vi "AlliGator Lifetime Variance Maps Calculation.vi"(7 "AlliGator Ctrl Refnums":T3, 8 "error in (no error)":errorcluster, 9 "Function Parameters":T1={"Function"=enum."Single-Exponential", "Amplitude"=0.0, "Exponent/Scale"=0.0, "Baseline"=0.0, "Residuals SDV"=0.0, "Minimum CL (%)"=1.0, "Analysis Type"=enum."Reference", "Bootstrap SDV x Scale Factor"=1.0, "Residuals SDV x Scale Factor"=1.0, "Low CL Percentile to Reject (%)"=1.0} {"Low CL Percentile to Reject (%)" min=0.0 max=100.0; "Residuals SDV x Scale Factor" min=0.0 max=100.0; "Bootstrap SDV x Scale Factor" min=0.0 max=100.0; "Minimum CL (%)" min=1.0}, 11 "AlliGator IV DVR in":refnum<data-value>) -> (0 "error out":errorcluster, 1 "Parameter Map Names":string[](array[string]), 2 "New Parameter Set Name":string, 3 "AlliGator IV DVR out":refnum<data-value>, 4 "Message":string)   [LabVIEW 2021, in "AlliGator Decay Fit Parameter Map.lvlib"]
uses:
  AlliGator Decay Fit Parameter Map.lvlib
  Internal Variables/AlliGator Internal Variables v2.ctl
  <vilib>/vision/Image Controls.llb/IMAQ Image.ctl
  Internal Variables/AlliGator Gate Image Set.ctl
  Files/AlliGator FLI Dataset Type.ctl
  Files/AlliGator Data Series Type.ctl
  Dual-Channel Datasets/AlliGator Dataset Channel.ctl
  Settings/AlliGator Gate Arithmetic.ctl
  Source Image/AlliGator Displayed Image.ctl
  Image/Named ROI Description.ctl
  Phasor Graph/AlliGator Decay Metadata v3.ctl
  Decay Analysis/Decay Preprocessing/AlliGator Decay Background Subtraction Info.ctl
  Decay Analysis/Decay Preprocessing/AlliGator Baseline Subtraction Method.ctl
  Graphs/XY Graph/XY Graph Plot Shift Parameters.ctl
  Graphs/XY Graph/XY Graph Plot Shift Method.ctl
  Decay Analysis/Decay Preprocessing/AlliGator Decay Extrapolation Parameters.ctl
  Phasor/Calibration Phasor (m, phi).ctl
  Phasor/Phasor Reference Series.ctl
  Phasor/Phasor Calibration Map v2.ctl
  Phasor/Phasor (g, s).ctl
  Phasor Graph/AlliGator Raw Phasor Plot Data v5.ctl
  Phasor/Phasor Standard Deviation Options.ctl
  Phasor Plot/AlliGator Phasor Multi-Harmonic Data.ctl
  Phasor/Phasor Harmonic Data.ctl
  AlliGator Decay Fit Options & Parameters v4.ctl
  Fits/IRF(X)PSED/Decay Fit Options v4.ctl
  Fits/Decay Convolution/Decay Model.ctl
  Fits/Residual Type.ctl
  Fits/IRF(X)PSED/Fit Weights Type v2.ctl
  Fits/Non-linear Fitting Method v2.ctl
  Fits/Fit Calculation Method.ctl
  Fits/Non-linear Fitting Algorithm.ctl
  Decay Analysis/Decay Fit/AlliGator Decay Fit Parameter Constraints 2.ctl
  Fits/IRF(X)PSED/Decay Fit Parameters In List.ctl
  Fits/IRF(X)PSED/MLE Baseline Offset Type.ctl
  Decay Analysis/Decay Preprocessing/AlliGator Decay Preprocessing Parameters.ctl
  Fits/IRF(X)PSED/Decay Fit Parameters & Derived Quantities List v2.ctl
  Fits/IRF(X)PSED/Decay Fit Result Constraint.ctl
  AlliGator Parameter Maps Data.ctl
  GUI/AlliGator Ctrl Refnums.ctl
  GUI/AlliGator Other Ctrl Refnums.ctl
  GUI/AlliGator State Indicator.ctl
  GUI/AlliGator Main Window Tabs.ctl
  GUI/AlliGator Phasor Plot Ctrl Refnums.ctl
  GUI/AlliGator Phasor Graph Ctrl Refnums.ctl
  Phasor/Phasor Calibration Type.ctl
  GUI/AlliGator Dataset Ctrl Refnums.ctl
  GUI/AlliGator Registered Events Ctrl Refnums.ctl
  GUI/AlliGator Image Histogram Control Refnums.ctl
  Histograms/Linear Histogram Options.ctl
  Histograms/Histogram Bin Option.ctl
  Histograms/Histogram Bin Position.ctl
  AlliGator Decay Fit Map Control Refnums.ctl
  Parameter Map/AlliGator Parameter Map Control Refnums.ctl
  AlliGator Function Parameters.ctl
  AlliGator CV(tau) Model Function.ctl
  Globals, Variables, Constants/AlliGator Variables List.ctl
  Camera Noise Influence on Lifetime/Lifetime Variance Data.ctl
  Variant/Variant to Data/Variant to U16.vi
  Variant/Variant to Data/Variant to I32.vi
  <vilib>/Utility/error.llb/Error Cluster From Error Code.vi
  <vilib>/ErrorRing/Error Ring.xnode
  Globals, Variables, Constants/AlliGator Globals, Variables & Constants.lvlib
  Variant/Variant to Data/Variant to Data.lvlib
  Files/AlliGator Files.lvlib
  Fits/Fits.lvlib
  Image/Image.lvlib
  Lifetime & Other Parameters/AlliGator Lifetime & Other Parameters.lvlib
  Strings/Strings.lvlib
  Time/Time.lvlib
  Variant/Variant.lvlib
  Phasor/Phasor.lvlib
  Decay Analysis/Decay Preprocessing/AlliGator Decay Preprocessing.lvlib
  Phasor Graph/AlliGator Phasor Graph.lvlib
  Internal Variables/AlliGator Internal Variables.lvlib
  Phasor Plot/AlliGator Phasor Plot.lvlib
  Source Image/AlliGator Source Image.lvlib
  Decay Analysis/Decay Fit/AlliGator Decay Fit.lvlib
  Settings/AlliGator Settings.lvlib
  Dual-Channel Datasets/AlliGator Dual-Channel Datasets.lvlib
  GUI/AlliGator GUI.lvlib
  Histograms/Histogram Window.lvlib
  Graphs/XY Graph/XY Graph Add-Ons.lvlib
  Parameter Map/AlliGator Parameter Map.lvlib
panel:
  out "CPU (s)":dbl
  # "see the AlliGator License on the block diagram (Ctrl+E or Window:Show Block Diagram)"
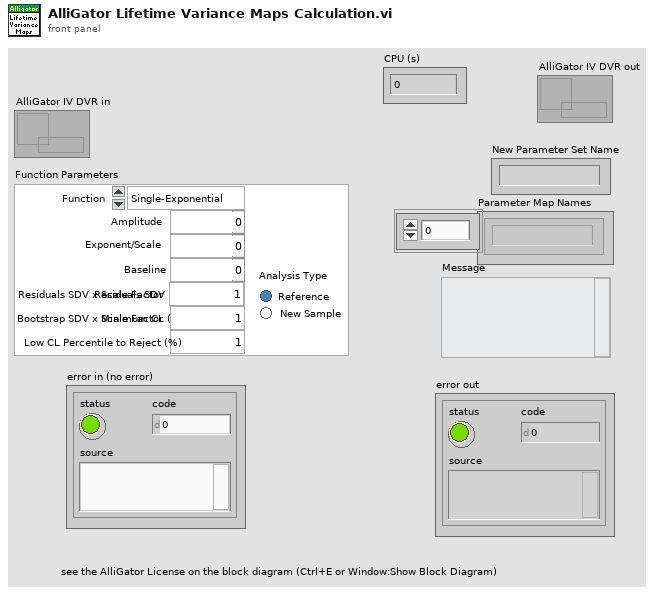
[diagram p1: front panel]
types:
  T1 = typedef "AlliGator Decay Fit Parameter Map.lvlib/AlliGator Function Parameters.ctl" = cluster{"Function":T2, "Amplitude":dbl, "Exponent/Scale":dbl, "Baseline":dbl, "Residuals SDV":dbl, "Minimum CL (%)":dbl, "Analysis Type":enum32{"Reference", "New Sample"}, "Bootstrap SDV x Scale Factor":dbl, "Residuals SDV x Scale Factor":dbl, "Low CL Percentile to Reject (%)":dbl}
  T2 = typedef "AlliGator Lifetime & Other Parameters.lvlib/AlliGator CV(tau) Model Function.ctl" = enum16{"Single-Exponential", "Power Law"}
  T3 = typedef "AlliGator GUI.lvlib/AlliGator Ctrl Refnums.ctl" = cluster{"Other AlliGator Ctrl Refnums":T4, "Phasor Plot Ctrl Refnums":T5, "Phasor Graph Ctrl Refnums":T6, "Dataset Control Refnums":T7, "Registered Events Ctrl Refnums":T8, "Image Histogram Ctrl Refnums":T9, "Decay Fit Map Ctrl Refnums":T10, "Parameter Map Ctrl Refnums":T11}
  T4 = typedef "AlliGator GUI.lvlib/AlliGator Other Ctrl Refnums.ctl" = cluster{"State Indicators":refnum<vi>, " Progress Bar":refnum<vi>, "Decay Graph Active":refnum<vi>, "Decay Statistics Bin":refnum<vi>, "Time Step":refnum<vi>, "Use File Timestamp":refnum<vi>, "Tab Control":refnum<vi>, "CPU":refnum<vi>, "Abort Fit":refnum<vi>, "Dataset File/Folder Path":refnum<vi>, "Abort ROI Creation":refnum<vi>, "Event LED":refnum<vi>, "Dataset File/Folder Path 2":refnum<vi>, "Dataset File/Folder Path 3":refnum<vi>, "Dataset File/Folder Path 4":refnum<vi>, "Dataset File/Folder Path 5":refnum<vi>, "Dataset File/Folder Path 6":refnum<vi>, "Dataset File/Folder Path 7":refnum<vi>, "Dataset File/Folder Path 8":refnum<vi>, "Dataset File/Folder Path 9":refnum<vi>, "Dataset File/Folder Path 10":refnum<vi>, "Dataset File/Folder Path 11":refnum<vi>}
  T5 = typedef "AlliGator GUI.lvlib/AlliGator Phasor Plot Ctrl Refnums.ctl" = cluster{"Phasor Ratio":refnum<vi>, "Modulus Lifetime":refnum<vi>, "Phasor at cursor (m, phi)":refnum<vi>, "Phase Lifetime":refnum<vi>, "Phasor at cursor (g, s)":refnum<vi>, "Phasor Plor Average Lifetime":refnum<vi>, "Phasor Plot Active":refnum<vi>, "Save Phasor Plot":refnum<vi>, "Image Overlay Color":refnum<vi>, "Phasor Plot Color Scale":refnum<vi>, "Reference 1 Button":refnum<vi>, "Reference 2 Button":refnum<vi>, "True Phasor Plot Value":refnum<vi>}
  T6 = typedef "AlliGator GUI.lvlib/AlliGator Phasor Graph Ctrl Refnums.ctl" = cluster{"Phasor Ratio":refnum<vi>, "Modulus Lifetime":refnum<vi>, "Phasor at cursor (m, phi)":refnum<vi>, "Phase Lifetime":refnum<vi>, "Phasor at cursor (g, s)":refnum<vi>, "Phasor Graph Average Lifetime":refnum<vi>, "Phasor Graph Active":refnum<vi>, "Save Phasor Graph":refnum<vi>, "Phasor Frame Slide":refnum<vi>, "Single Step Phasor":refnum<vi>, "Calibration Type":refnum<vi>, "Show Line":refnum<vi>, "Phase Lifetime 1":refnum<vi>, "Phase Lifetime 2":refnum<vi>, "Phasor Graph Frequency":refnum<vi>, "Phasor Reference 1 Control":refnum<vi>, "Phasor Reference 2 Control":refnum<vi>, "Calibration Lifetime":refnum<vi>, "Phase Lifetime SDV":refnum<vi>, "Average Lifetime SDV":refnum<vi>, "Phasor Ratio SDV":refnum<vi>, "Modulus Lifetime SDV":refnum<vi>}
  T7 = typedef "AlliGator GUI.lvlib/AlliGator Dataset Ctrl Refnums.ctl" = cluster{"Current Data":refnum<vi>, "Gate Image Slide":refnum<vi>, "Time Point Slide":refnum<vi>, "Current Time Stamp":refnum<vi>, "Save Image":refnum<vi>, "Displayed Image":refnum<vi>, "Overlay Mode":refnum<vi>, "Phasor Overlay Color":refnum<vi>, "Image Color Scale":refnum<vi>, "Use ROI as Search Area":refnum<vi>, "Source Image ROI Color":refnum<vi>, "True Pixel Value":refnum<vi>}
  T8 = typedef "AlliGator GUI.lvlib/AlliGator Registered Events Ctrl Refnums.ctl" = cluster{"Time Point Slider":refnum<vi>, "Phasor Plot Display Range":refnum<vi>, "Decay Graph":refnum<vi>, "Decay Statistics Graph":refnum<vi>, "Intensity Time Trace":refnum<vi>, "Phasor Graph":refnum<vi>, "Phasor Ratio Graph":refnum<vi>, "Lifetime Graph":refnum<vi>, "Phasor Plot Display":refnum<vi>, "Source Image Display":refnum<vi>, "Decay Fit Parameter Map Display Range":refnum<vi>, "Decay Fit Parameter Map Display":refnum<vi>, "Parameter Map Display Range":refnum<vi>, "Parameter Map Display":refnum<vi>, "Phasor Plot Display Range":refnum<vi>}
  T9 = typedef "AlliGator GUI.lvlib/AlliGator Image Histogram Control Refnums.ctl" = cluster{"Image Histogram":refnum<vi>, "Image Histogram Options":refnum<vi>, "Image Histogram Active":refnum<vi>, "Image Histogram Upper Percentile":refnum<vi>, "Image Histogram Lower Percentile":refnum<vi>, "Auto-Adjust Contrast":refnum<vi>}
  T10 = typedef "AlliGator Decay Fit Parameter Map.lvlib/AlliGator Decay Fit Map Control Refnums.ctl" = cluster{"Decay Fit Parameter Map Color Scale":refnum<vi>, "Decay Fit Parameter":refnum<vi>, "Max Parameter":refnum<vi>, "Min Parameter":refnum<vi>, "Decay Fit Parameter Map Display":refnum<vi>, "Decay Fit Parameter Map Display Range":refnum<vi>, "Decay Parameter Map X":refnum<vi>, "Decay Parameter Map Y":refnum<vi>, "Decay Parameter Map Value":refnum<vi>}
  T11 = typedef "AlliGator Parameter Map.lvlib/AlliGator Parameter Map Control Refnums.ctl" = cluster{"Parameter Map Color Scale":refnum<vi>, "Map Parameter":refnum<vi>, "Max Parameter":refnum<vi>, "Min Parameter":refnum<vi>, "Parameter Map Display":refnum<vi>, "Parameter Map Display Range":refnum<vi>, "Parameter Map Set":refnum<vi>, "Parameter Map X":refnum<vi>, "Parameter Map Y":refnum<vi>, "Parameter Map Value":refnum<vi>}
  T12 = typedef "AlliGator Globals, Variables & Constants.lvlib/AlliGator Variables List.ctl" = enum16{"---- GUI ----", "GUI:Initialization Status", "GUI:State Indicators Refnum", "GUI:Original AlliGator Menu Items", "GUI:Current Action Loop State", "GUI:Script in progress", "GUI:Playback", "GUI:Loop Playback", "GUI:Search ROI Used", "GUI:Search ROI", "Decay Graph Max Legend Size", "Intensity Graph Max Legend Size", "Decay Statistics Graph Max Legend Size", "Phasor Graph Max Legend Size", "Phasor Ratio Graph Max Legend Size", "Lifetime Graph Max Legend Size", "---- Files ----", "Files:Export Dataset Frames as Individual Files", "Files:Show Batch Export Help Balloons", "Files:Frames in Dataset", "Files:ptu File Frame Start Indices", "Files:Current Frame in Dataset", "Files:Current Frame Timestamp", "Files:Dataset Loaded", "Files:Dataset Metadata", "Files:Dataset Channel", "Files:Dataset Data Description", "Files:Background Dataset Metadata", "Files:Background Dataset Channel", "Files:Background Dataset Data Description", "Files:Background File Subtraction", "Files:Background File Path", "Files:Background File Pile-up Correction", "Files:Background File Pixel Well Capacity", "Files:Background File Scaling Factor", "Files:Current Dataset Load Settings", "Files:Dataset Path", "Files:ICCD-specific Information", "Files:Macrotime Gate Separation", "------ Python Plugins ------", "Python Plugins:Information", "Python Plugins:Python Session", "Python Plugins:Valid Python Session?", "---- Source Image ----", "Source Image:ROIs", "Source Image:Current ROI", "Source Image:ROI Event Refnum", "X_Source Image:Display Range", "X_Source Image:Palette Information", "X_Source Image:Type of Displayed Image", "X_Time Gate Slider", "Source Image:Palette List", "Source Image:Scale", "Source Image:ROI Overlay Color", "Source Image:Overlay to Erase", "Source Image:Is Displayed Image Accumulated", "Source Image:White Light Image Modified", "Source Image:Mask Image Modified", "---- Image Profile Window ----", "Image Profile:Window Event Refnum", "Image Profile:IntensityType", "Image Profile:Intensity Average Type", "Image Profile:Intensity-weighted SDV", "Image Profile:Box Profile Type", "Image Profile:Window Open", "Image Profile:Plotted Fit Parameter", "------ Phasor Graph -------", "Phasor Graph:Show Line", "---- Phasor Plot ---", "Phasor Plot:Parameters Changed", "Phasor Plot:FLI Dataset Modified since last Calculation", "Phasor Harmonics Data", "Selected Phasor Harmonics", "Phasor Harmonic Manager Event Refnum", "Phasor Plot:ROIs", "Phasor Plot:Current ROI", "Phasor Plot:ROI Event Refnum", "Phasor Plot:Image Reference Points", "Phasor Plot:Computed", "Phasor Plot:Palette Information", "Phasor Plot:Palette List", "Phasor Plot:Phasor Ratio Palette Information", "Phasor Plot:Phasor Ratio Palette List", "Phasor Plot:Image Scale", "Phasor Plot:Image Overlay to Erase", "Phasor Plot:Image Elements to Update", "Phasor Plot:Current Calculation Parameters", "Phasor Plot:Current Calibration Options", "Phasor Plot:Reset Cumulated Phasor Plot", "Phasor Plot:Reference 1", "Phasor Plot:Lifetime Reference 1", "Phasor Plot:Reference 1 Frequency", "Phasor Plot:Reference 2", "Phasor Plot:Lifetime Reference 2", "Phasor Plot:Reference 2 Frequency", "---- Decay Analysis ----", "Number of Selected Decays to Fit", "LS Fit Results", "LAR Fit Results", "BS Fit Results", "Last Decay Max - Min", "Best Fit Parameters", "Best Fit Parameter Names", "Actual Size X", "Actual Size Y", "Binning X", "Binning Y", "Actual # Gates", "Dataset Number", "Gates to...", "Gates Skipped", "Gates to keep", "Gate Step", "Gate Separation", "Reversed Gates", "Pile-up Correction", "Pixel Well Capacity", "Background Subtracted", "Background Subtraction Method", "Background Definition Range", "Background File (deprecated)", "Number of Dataset Accumulated", "Array of Accumulated Dataset Paths", "Do Averaged Datasets", "Destination File Path", "Process Plot Target", "Use 1/D as Phasor Frequency", "---- Decay Fit Parameter Map -----", "Decay Fit Parameter Map:Palette Information", "Decay Fit Parameter Map:Palette List", "Decay Fit Parameter Map:X Resolution", "Decay Fit Parameter Map:Y Resolution", "Decay Fit Parameter Map:Use Decay Fit Result Constraints", "Decay Fit Parameter Map:Decay Fit Result Constraints", "Decay Fit Parameter Map:Decay Fit Result Constraints Applied", "---- Parameter Map ----", "Parameter Map:Palette Information", "Parameter Map:Palette List", "------- Local Decay Window ---------", "Local Decay Graph Window:Event Refnum", "Local Decay Graph Window:Use normalized IRF for convolution", "----- Miscellaneous ----", "Misc:Skippable Dialog Windows Status"}
  T13 = typedef "Image.lvlib/Named ROI Description.ctl" = cluster{"ROI Descriptor":T14, "ROI Name":string, "Overlay Color":u32}
  T14 = typedef "ROI Descriptor" = cluster{"Global Rectangle":i32[], "Contours":cluster{"ID":enum32{"External", "Internal"}, "Type":u32, "Coordinates":i32[]}[]}
  T15 = typedef "Fits.lvlib/Decay Fit Parameters & Derived Quantities List v2.ctl" = enum16{"Offset", "Baseline", "A_1", "tau_1", "A_2", "tau_2", "<tau>_a", "f1_a", "f2_a", "<tau>_i", "f1_i", "f2_i", "-", "R^2", "Chi^2"}
  T16 = typedef "AlliGator Decay Fit Parameter Map.lvlib/AlliGator Parameter Maps Data.ctl" = cluster{"Map Set Name":string, "[Parameter Names]":string[], "[[Parameters]]":dbl[][], "[[Parameter SDVs]]":dbl[][], "Decay Array Time Axis":dbl[], "[[IRFs]]":dbl[][], "IRF Array Time Axis":dbl[], "X Resolution":i32, "Y Resolution":i32, "Intensity Array":dbl[]}
  T17 = typedef "AlliGator Decay Fit Parameter Map.lvlib/Lifetime Variance Data.ctl" = cluster{"ROI Name":string, "Intensity Array":sgl[], "Lifetime Array":dbl[], "Coordinate Array":cluster{"X":i32, "Y":i32}[], "I Slice Bin Boundaries":dbl[], "Sliced <tau>":dbl[], "Sliced SDV(<tau>)":dbl[], "Sliced CV(<tau>)":dbl[], "Sliced #Elements":i32[], "I Slice <I>":dbl[], "Sliced CV SDV(<tau>)":dbl[]}
  T18 = typedef "AlliGator Internal Variables.lvlib/AlliGator Internal Variables v2.ctl" = cluster{"----------------------------- Images -----------------------------":u8, "Displayed Image":T19, "White Light Image":T19, "Mask Image":T19, "ROI Mask Image":T19, "Current Dataset Images 1":T20, "Background Dataset Images 1":T20, "Current Dataset Images 2":T20, "Background Dataset Images 2":T20, "Current Dataset Arithmetic Images":T20, "Accumulated Dataset Images 1":T20, "Accumulated Dataset Images 2":T20, "Accumulated Dataset Arithmetic Images":T20, "----------------------------- File Paths -----------------------------":u8, "Phasor Plot Image":T19, "Decay Fit Parameter Map Image":T19, "Parameter Map Image":T19, "Single Data Point Path":path, "White Light Image Path":path, "Mask Image Path":path, "Time-Series Folder":path, "[Time-Series Paths]":path[], "----------------------------- FLI Dataset -----------------------------":u8, "Current Dataset":i32, "Single Dataset Type":T21, "Current Folder":string, "AlliGator Data Series Type":T22, "# Datasets":i32, "Dual-Channel Dataset":bool, "Selected Channel Name":string, "Dataset Channel":T23, "Channel Arithmetic":T24, "Dual-Channel Background Dataset":bool, "Background Channel":T23, "Dual-Channel Accumulated Dataset":bool, "Start Time":dbl, "[Time-Series Timestamps]":dbl[], "[Intensity Corrections]":dbl[], "Time Series Script":bool, "Type of Displayed Image":T25, "Gate Image Slide":u16, "# Gates":i32, "ROIs":T13[], "----------------------------- Decays -----------------------------":u8, "ROI Decay":cluster{"t Array":dbl[], "I Array":dbl[]}, "Valid Decay":bool, "Decay  Metadata":T26, "Reference Decay Plot Name":string, "Reference Decay":cluster{"t Array":dbl[], "I Array":dbl[]}, "Decay Shift Plot":cluster{"Time Stamps":dbl[], "Decay Shifts":dbl[]}, "[Decays Max Values]":sgl[], "[Decays Min Values]":sgl[], "----------------------------- Calibration -----------------------------":u8, "Calibration Phasor":T32, "Calibration Phasor Series":T33, "Phasor Calibration Map":T34, "Calibration Map MD5 Digest":string, "----------------------------- Phasor Graph -----------------------------":u8, "Last Raw Phasor":T35, "Last Calibrated Phasor":T35, "Last Calibrated Phasor SDV":T35, "Phasor Graph:Phasor Plot":cluster{"g Array":dbl[], "s Array":dbl[]}, "Phasor Graph:Phasor SDV Plot":cluster{"g Array":dbl[], "s Array":dbl[]}, "[Phasor Graph:Raw Phasor Plots]":T36[], "Phasor Plot locked to Ref 1":i32, "[Phasor Plot(s) locked to Ref 1]":i32[], "[Phasor Plot(s) locked to Ref 2]":i32[], "[Pixel Phasors]":T35[], "----------------------------- Phasor Plot -----------------------------":u8, "[[Sum Image]]":dbl[][], "[[CSG Phasors]]":csg[][], "[[Valid Pixel?]]":bool[][], "[[Phasor Ratios]]":dbl[][], "[[Average Lifetimes]]":dbl[][], "Amplitude Weighted Average Lifetime":bool, "I/m/phi Dataset":cluster{"I/m/phi Dataset?":bool, "Base Frequency":dbl[unit], "Harmonic Orders":u8[]}, "Multi Phasor Plot Data":T38, "----------------------------- Decay Fit Parameter Map -----------------------------":u8, "Decay Fit Options & Parameters":T40, "Fit Options: Decay Preprocessing Parameters":T51, "Fit Options: Reference Decay":cluster{"t Array":dbl[], "I Array":dbl[]}, "Is Full Image Parameters Map":bool, "Is Single-Pixels Parameters Map":bool, "NLSF Parameters Map X Resolution":i32, "NLSF Parameters Map Y Resolution":i32, "[Single Decay Fit Parameters]":dbl[], "Fit Model":T42, "[[Multiple Decays Fit Parameters]]":dbl[][], "[[Multiple Decays Fit Parameter SDVs]]":dbl[][], "[[IRFs]]":dbl[][], "[ROI Descriptors]":T14[], "IRF Array Time Axis":dbl[], "Decay Array Time Axis":dbl[], "[Decay Fit Parameter Names]":T15[], "[Decay Sum]":dbl[], "Array of Decay Fit Result Constraints":T52[], "Selected ROIs Array":bool[], "----------------------------- Parameter Maps -----------------------------":u8, "[Map Set Names]":string[], "[Parameter Maps]":T16[], "[[User-defined Quantities]]":dbl[][], "User-defined Quantity":string}
  T19 = typedef "IMAQ Image.ctl" = refnum<image>
  T20 = typedef "AlliGator Internal Variables.lvlib/AlliGator Gate Image Set.ctl" = cluster{"SGL Gate Images":T19[], "SGL Sum Image":T19, "SGL Max Image":T19, "SGL Min Image":T19}
  T21 = typedef "AlliGator Files.lvlib/AlliGator FLI Dataset Type.ctl" = enum16{"HDF5 FLI Dataset", "Gate Image Folder", ".sdt FLI Dataset (Becker & Hickl)", ".ptu FLI Dataset (PicoQuant)", "SS1 FLI Dataset", "SS2 FLI Dataset", "I/m/phi Dataset", ".bin FLI Dataset (PicoQuant Binned)", ".bin FLI Dataset (Piccolo Binned)", ".mat FLI Dataset"}
  T22 = typedef "AlliGator Files.lvlib/AlliGator Data Series Type.ctl" = enum16{"Not a Supported Series", "Gate Images Folder Series", "SwissSPAD 2 Dataset Series", "B&H FLI Dataset Series", "PicoQuant PTU FLI Dataset Series", "PicoQuant BIN FLI Dataset Series", "Piccolo hist BIN FLI Dataset Series", "HDF5 FLI Dataset Series"}
  T23 = typedef "AlliGator Dual-Channel Datasets.lvlib/AlliGator Dataset Channel.ctl" = enum16{"G2", "INT"}
  T24 = typedef "AlliGator Settings.lvlib/AlliGator Gate Arithmetic.ctl" = enum16{"None", "INT-G2", "G2/INT*<INT>", "(1 - G2/INT)*<INT>"}
  T25 = typedef "AlliGator Source Image.lvlib/AlliGator Displayed Image.ctl" = enum16{"Single Gate", "Sum of All Gates", "Max of All Gates", "Min of All Gates", "-", "White Ligth Image", "Mask Image"}
  T26 = typedef "AlliGator Phasor Graph.lvlib/AlliGator Decay Metadata v3.ctl" = cluster{"ROI Descriptor":T14, "ROI Center":cluster{"X":i32, "Y":i32}, "Decay Background Subtraction Info":T27, "Decay Reverted":bool, "Decay Smoothened":bool, "Decay Straightened":bool, "Fitted Tau (Decay Straightening)":dbl, "Decay Shift Parameters":T29, "Decay Shifted":bool, "Decay Extrapolated":bool, "Decay Extrapolation Parameters":T31, "Decay Normalized":bool, "Fold Decay":bool, "# Folds":u32}
  T27 = typedef "AlliGator Decay Preprocessing.lvlib/AlliGator Decay Background Subtraction Info.ctl" = cluster{"Laser Period":dbl[unit], "Gate Duration":dbl[unit], "Baseline Subtraction Method":T28, "Background Definition Range":cluster{"Min Gate":dbl[unit], "Max Gate":dbl[unit]}, "Total Intensity w/o Bkgd Subtraction":dbl, "Bkgd-subtracted Intensity (exp)":dbl, "# Data Points":i32, "Background/Gate":dbl, "Fitted Lifetime":dbl[unit], "Bkgd-subtracted Intensity (theo)":dbl}
  T28 = typedef "AlliGator Decay Preprocessing.lvlib/AlliGator Baseline Subtraction Method.ctl" = enum16{"Mean", "Min", "Square Gated Single-Exponential", "File", "Constant"}
  T29 = typedef "XY Graph Add-Ons.lvlib/XY Graph Plot Shift Parameters.ctl" = cluster{"Type":T30, "Shift":dbl[unit], "Threshold":dbl, "Rotate":bool}
  T30 = typedef "XY Graph Add-Ons.lvlib/XY Graph Plot Shift Method.ctl" = enum16{"Default", "CFD", "Threshold", "Cross-Correlation"}
  T31 = typedef "AlliGator Decay Preprocessing.lvlib/AlliGator Decay Extrapolation Parameters.ctl" = cluster{"Additional Points":u32, "Head Fraction":dbl, "Fitted Tau":dbl, "Use Periodicity":bool, "Use Cursors":bool, "Tail Fraction":dbl}
  T32 = typedef "Phasor.lvlib/Calibration Phasor (m, phi).ctl" = cluster{"m":dbl, "phi":dbl, "Phasor Frequency":dbl[unit], "Reference Lifetime":dbl[unit]}
  T33 = typedef "Phasor.lvlib/Phasor Reference Series.ctl" = cluster{"m Array":dbl[], "phi Array":dbl[], "Phasor Frequency":dbl[unit], "Calibration Lifetime":dbl[unit]}
  T34 = typedef "Phasor.lvlib/Phasor Calibration Map v2.ctl" = cluster{"Phasor Frequency":dbl[unit], "Calibration Lifetime":dbl[unit], "ROI Centers":cluster{"X":i32, "Y":i32}[], "ROI Descriptors":T14[], "Map Resolution X":i32, "Map Resolution Y":i32, "z Array":cdb[]}
  T35 = typedef "Phasor.lvlib/Phasor (g, s).ctl" = cluster{"g":dbl, "s":dbl}
  T36 = typedef "AlliGator Phasor Graph.lvlib/AlliGator Raw Phasor Plot Data v5.ctl" = cluster{"Phasor Plot Name":string, "Raw Phasor Plot":T35[], "Phasor Frequency":dbl[unit], "[Decay Metadata]":T26[], "Raw Phasor Plot SDV":T35[], "Phasor SDV Options":T37, "[Calibration Phasor]":T32[], "Intensity Array":dbl[]}
  T37 = typedef "Phasor.lvlib/Phasor Standard Deviation Options.ctl" = cluster{"Compute Estimated SDV":bool, "# Replicas":u32, "Use Estimated Average Phasor":bool}
  T38 = typedef "AlliGator Phasor Plot.lvlib/AlliGator Phasor Multi-Harmonic Data.ctl" = cluster{"Base Frequency":dbl[unit], "# Harmonics":u8, "Harmonic Orders":u8[], "Phasor Plot Settings Checksum":u64, "Phasor Harmonic Data Array":T39[]}
  T39 = typedef "Phasor.lvlib/Phasor Harmonic Data.ctl" = cluster{"Phasor Harmonic Name":string, "Phasor Plot Settings Checksum":u64, "Phasor Frequency":dbl[unit], "Base Frequency":dbl[unit], "Harmonic Order":u8, "Phasor Plot Parameters":string, "Phasor Array [[CSG]]":csg[][], "Dataset File Path":path}
  T40 = typedef "AlliGator Decay Fit Parameter Map.lvlib/AlliGator Decay Fit Options & Parameters v4.ctl" = cluster{"SYNC Period":dbl[unit], "Fit Options":T41, "Fit Parameter Constraints":T48[], "MLE Baseline Offset":dbl, "MLE Baseline Offset Type":T50}
  T41 = typedef "Fits.lvlib/Decay Fit Options v4.ctl" = cluster{"Show Fit Residuals":bool, "Fit Model":T42, "Residual Type":T43, "Max Decay Percentile":dbl, "Min Decay Percentile":dbl, "Show Full Decay":bool, "Weights":T44, "Fitting Method":T45, "Compute Parameter Uncertainties":bool, "Periodic Boundaries":bool, "Model Calculation":T46, "Period":dbl[unit], "Termination Criteria":cluster{"Max Iterations":i32, "Max Function Calls":i32, "Max Time":dbl[unit], "Function Tolerance":dbl, "Parameter Tolerance":dbl, "Gradient Tolerance":dbl, "Min Lambda":dbl, "Max Lambda":dbl, "Initial Tick Count":u32}, "Offset Resolution":dbl[unit], "Use Local IRF":bool, "Fitting Algorithm":T47, "Show Confidence Interval ":bool, "Confidence Level":dbl}
  T42 = typedef "Fits.lvlib/Decay Model.ctl" = enum16{"1-Exponential", "2-Exponentials"}
  T43 = typedef "Fits.lvlib/Residual Type.ctl" = enum16{"Standard", "Normalized", "Reduced"}
  T44 = typedef "Fits.lvlib/Fit Weights Type v2.ctl" = enum16{"Unweighted", "1/Variance (Neyman)", "1/Variance (Pearson)", "Best of All"}
  T45 = typedef "Fits.lvlib/Non-linear Fitting Method v2.ctl" = enum16{"Least Square", "Least Absolute Residual", "Bisquare", "MLE", "-", "Best of All"}
  T46 = typedef "Fits.lvlib/Fit Calculation Method.ctl" = enum16{"Simulation", "Convolution", "Integration"}
  T47 = typedef "Fits.lvlib/Non-linear Fitting Algorithm.ctl" = enum16{"Levenberg-Marquardt", "Trust-Region Dogleg"}
  T48 = typedef "AlliGator Decay Fit.lvlib/AlliGator Decay Fit Parameter Constraints 2.ctl" = cluster{"Fit Parameter":T49, "Min Value":dbl, "Max Value":dbl, "Global":bool, "Used":bool}
  T49 = typedef "Fits.lvlib/Decay Fit Parameters In List.ctl" = enum16{"Offset", "Baseline", "A_1", "tau_1", "A_2", "tau_2"}
  T50 = typedef "Fits.lvlib/MLE Baseline Offset Type.ctl" = enum32{"Absolute", "Percentage"}
  T51 = typedef "AlliGator Decay Preprocessing.lvlib/AlliGator Decay Preprocessing Parameters.ctl" = cluster{"Background Subtraction":bool, "Straighten Decay":bool, "Reverse Gates":bool, "1-Normalized Decay":bool, "Smoothen Decay":bool, "Smoothing Parameter":dbl, "Shift Decay":bool, "Decay Shift Parameters":T29, "Extrapolate Decay":bool, "Additional Points":u32, "Head Fraction":dbl, "Pixel-Normalize Decay":bool, "Use Periodicity":bool, "Use Cursors":bool, "Tail Fraction":dbl, "Use Decay Pre-Processing":bool, "Fold Decay":bool, "# Folds":u32, "[0-1]-Normalized Decay":bool}
  T52 = typedef "Fits.lvlib/Decay Fit Result Constraint.ctl" = cluster{"Fit Parameter":enum16{"Offset", "Baseline", "A_1", "tau_1", "A_2", "tau_2", "<tau>_a", "f1_a", "f2_a", "<tau>_i", "f1_i", "f2_i", "-", "R^2", "Chi^2", "Max Relative Residual", "<Residual ACF>", "Residual ACF SDV", "tau_2/tau_1"}, "Min Value":dbl, "Max Value":dbl, "Use Constraint":bool}
  T53 = typedef "XY Graph Add-Ons.lvlib/XY Graph Sliced Mean & SDV Step Definition.ctl" = cluster{"Axis Start":dbl, "Axis Stop":dbl, "# Steps":i32, "Step Size":dbl, "Step Definition":T54, "Upper Percentile":dbl, "Lower Percentile":dbl, "Min # Data Points/Slice":i32, "Output Abscissa Statistics Plots":bool, "Bin Location":T55, "# Elements":i32, "Bootstrap CV's SDV":bool, "# Replicas":i32}
  T54 = typedef "AlliGator Lifetime & Other Parameters.lvlib/AlliGator Intensity Slice Definition.ctl" = enum32{"# Steps", "Step Size", "# Elements"}
  T55 = typedef "XY Graph Add-Ons.lvlib/XY Graph Sliced CV Abscissa Location.ctl" = enum16{"Left", "Center", "Mean", "Right"}
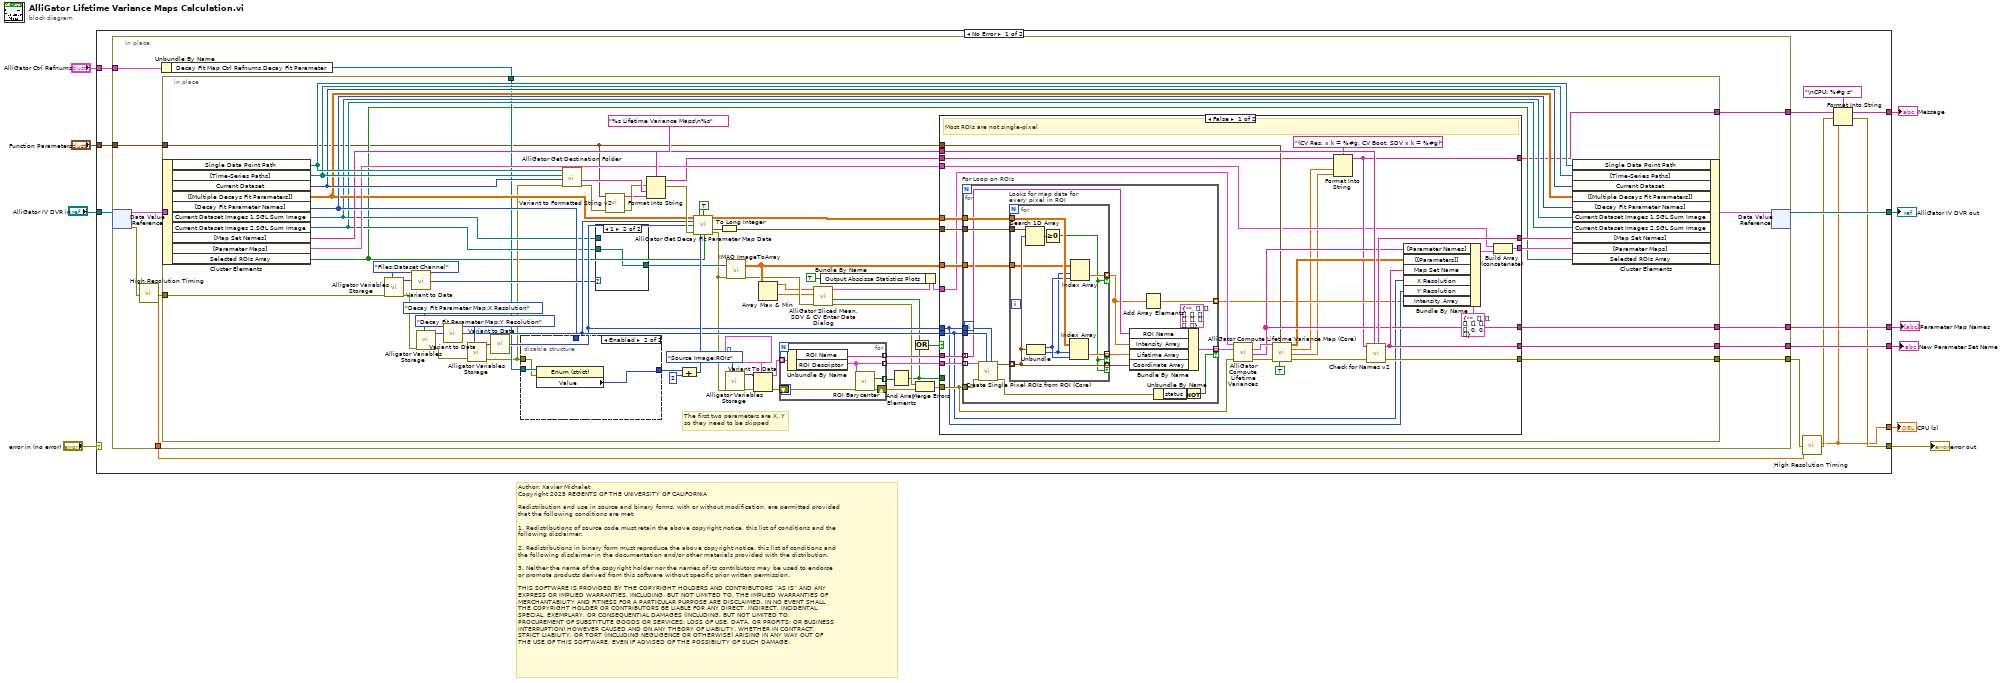
[diagram p0: block diagram]
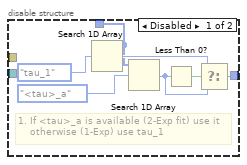
[diagram p2: hidden frame]
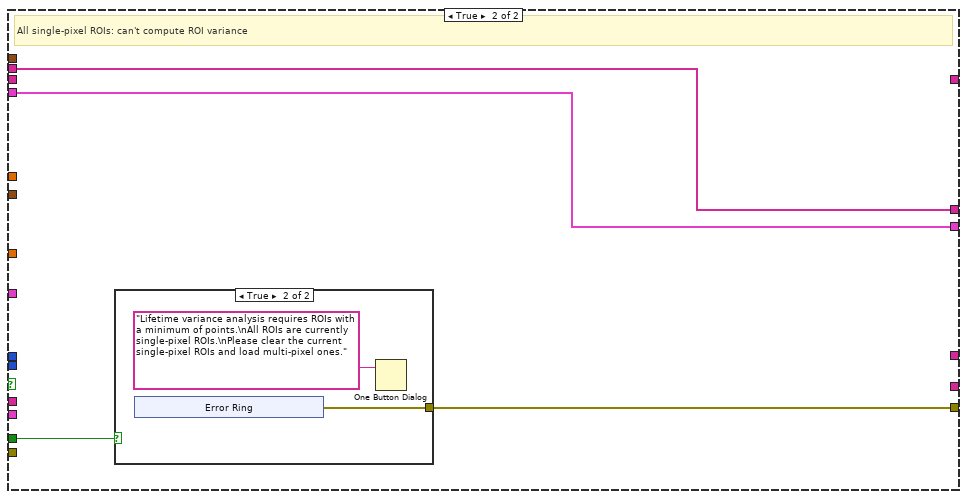
[diagram p3: hidden frame]
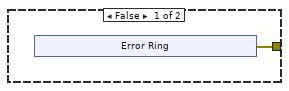
[diagram p4: hidden frame]
diagram:
  # "Author: Xavier Michalet\nCopyright 2025 REGENTS OF THE UNIVERSITY OF CALIFORNIA\n\nRedistribution and use in source and binary forms, with or without modification, are permitted provided\nthat the following conditions are met:\n\n1. Redistributions of source code must retain the above copyright notice, this list of conditions and the\nfollowing disclaimer.\n\n2. Redistributions in binary form must reproduce the above copyright notice, this list of conditions and\nthe following disclaimer in the documentation and/or other materials provided with the distribution.\n\n3. Neither the name of the copyright holder nor the names of its contributors may be used to endorse \nor promote products derived from this software without specific prior written permission.\n\nTHIS SOFTWARE IS PROVIDED BY THE COPYRIGHT HOLDERS AND CONTRIBUTORS “AS IS” AND ANY \nEXPRESS OR IMPLIED WARRANTIES, INCLUDING, BUT NOT LIMITED TO, THE IMPLIED WARRANTIES OF\nMERCHANTABILITY AND FITNESS FOR A PARTICULAR PURPOSE ARE DISCLAIMED. IN NO EVENT SHALL\nTHE COPYRIGHT HOLDER OR CONTRIBUTORS BE LIABLE FOR ANY DIRECT, INDIRECT, INCIDENTAL, \nSPECIAL, EXEMPLARY, OR CONSEQUENTIAL DAMAGES (INCLUDING, BUT NOT LIMITED TO, \nPROCUREMENT OF SUBSTITUTE GOODS OR SERVICES; LOSS OF USE, DATA, OR PROFITS; OR BUSINESS\nINTERRUPTION) HOWEVER CAUSED AND ON ANY THEORY OF LIABILITY, WHETHER IN CONTRACT, \nSTRICT LIABILITY, OR TORT (INCLUDING NEGLIGENCE OR OTHERWISE) ARISING IN ANY WAY OUT OF\nTHE USE OF THIS SOFTWARE, EVEN IF ADVISED OF THE POSSIBILITY OF SUCH DAMAGE."
  n1 = case shown="No Error" "error in (no error)" {
    selector: "error in (no error)" -> [_ w199]
    tunnel: "AlliGator Ctrl Refnums" -> [w22 _]
    tunnel: [w24 w198] -> w9
    tunnel: "AlliGator IV DVR in" -> [w23 w198]
    tunnel: [w13 w199] -> w7
    tunnel: "Function Parameters" -> [w21 _]
    tunnel: [w15 _] -> w4
    tunnel: [w12 _] -> w3
    tunnel: [w18 _] -> w2
    tunnel: [w17 _] -> w1
    frame No Error {
      n2 = in-place {
        in-place-border: w22 -> [w35]
        in-place-border: w21 -> [w32]
        in-place-border: [w31] -> w20
        in-place-border: [w29] -> w19
        in-place-border: [w27] -> w18
        in-place-border: [w26] -> w17
        in-place-border: [w25] -> w16
        n3 = in-place-dvr #1(w23) -> (w34:T18, w36:errorcluster)
        n4 = call "High Resolution Timing.vi"("Error In"=w36) -> ("elapsed (relative) seconds"=w29:dbl, "Error Out"=w30:errorcluster)  [unwired: 16 in, 1 out]
        n5 = Unbundle By Name(w35) -> ("Decay Fit Map Ctrl Refnums.Decay Fit Parameter"=w28:refnum<vi>)
        n6 = in-place {
          in-place-border: w34 -> [_]
          in-place-border: [w87] -> w25
          in-place-border: w30 -> [w76]
          in-place-border: [w54] -> w27
          in-place-border: [w52] -> w26
          in-place-border: w32 -> [w38]
          in-place-border: [w37] -> w31
          in-place-border: w28 -> [w45]
          w96 = TRUE ("Compute Decay Fit Parameter Map")
          # "The first two parameters are X, Y\nso they need to be skipped"
          n7 = in-place-cluster #2(w34) -> ("Single Data Point Path"=w61:path, "[Time-Series Paths]"=w60:path[], "Current Dataset"=w59:i32, "[[Multiple Decays Fit Parameters]]"=w51:dbl[][], "[Decay Fit Parameter Names]"=w58:T15[], "Current Dataset Images 1.SGL Sum Image"=w50:T19, "Current Dataset Images 2.SGL Sum Image"=w49:T19, "[Map Set Names]"=w55:string[], "[Parameter Maps]"=w53:T16[], "Selected ROIs Array"=w43:bool[])
          n8 = call "Alligator Variables Storage.vi"("AlliGator Variable"=AlliGator_Variables_List."Files:Dataset Channel" ("Alligator Variable"), "Error In"=w76) -> ("Error Out"=w75:errorcluster, "Data out"=w77:variant)  [unwired: 7 in, 1 out]
          n9 = call-poly "Variant to Data.vi"("Variant"=w77) -> ("U16 Value"=w74:u16)  [unwired: 8 in]
          n10 = call "Alligator Variables Storage.vi"("AlliGator Variable"=AlliGator_Variables_List."Decay Fit Parameter Map:X Resolution" ("Alligator Variable"), "Error In"=w75) -> ("Error Out"=w102:errorcluster, "Data out"=w101:variant)  [unwired: 7 in, 1 out]
          n11 = call-poly "Variant to Data.vi"("Variant"=w101) -> ("Value"=w84:i32)  [unwired: 8 in]
          n12 = call "Alligator Variables Storage.vi"("AlliGator Variable"=AlliGator_Variables_List."Decay Fit Parameter Map:Y Resolution" ("Alligator Variable"), "Error In"=w102) -> ("Error Out"=w44:errorcluster, "Data out"=w100:variant)  [unwired: 7 in, 1 out]
          n13 = call-poly "Variant to Data.vi"("Variant"=w100) -> ("Value"=w83:i32)  [unwired: 8 in]
          n14 = disable-structure shown="Enabled" {
            disable-tunnel: [w109 w113] -> w104
            disable-tunnel: w58 -> [w106 _]
            disable-tunnel: w45 -> [_ w115]
            disable-tunnel: w44 -> [_ w114]
            frame Disabled {
              # "1. If <tau>_a is available (2-Exp fit) use it\n    otherwise (1-Exp) use tau_1"
              n15 = Search 1D Array(1D array=w106, element=Decay_Fit_Parameters_&_Derived_Quantities_List_v2."tau_1") -> (index of element=w107:i32)  [unwired: 1 in]
              n16 = Search 1D Array(1D array=w106, element=Decay_Fit_Parameters_&_Derived_Quantities_List_v2."<tau>_a") -> (index of element=w110:i32)  [unwired: 1 in]
              n17 = Less Than 0?(x=w110) -> (x < 0?=w111:bool)
              n18 = Select(t=w107, s=w111, f=w110) -> (s? t:f=w109:i32)
            }
            frame Enabled {
              n19 = property class="Enum (strict)"(reference=w115, error in=w114) -> ("Value"=w113:T15)  [unwired: 2 out]
            }
          }
          n20 = call "AlliGator Get Destination Folder.vi"("Error In"=w44, "Current Data Set (-1: single)"=w59, "Time-Series Paths"=w60, "Single Data Point Path"=w61) -> ("Error Out"=w41:errorcluster, "Data Point Name"=w42:string)  [unwired: 4 in, 2 out]
          n21 = case shown="1" w74 {
            tunnel: w50 -> [w190 _]
            tunnel: w49 -> [_ w191]
            tunnel: [w190 w191] -> w73
            frame 0, Default {
            }
            frame 1 {
            }
          }
          n22 = call "Variant to Formatted String v2.vi"("error in (no error)"=w41, "Anything"=w38) -> ("error out"=w40:errorcluster, "String"=w39:string)  [unwired: 8 in]
          n23 = Format Into String(format string="%s Lifetime Variance Maps\n%s", error in=w40, w42, w39) -> (resulting string=w48:string, error out=w97:errorcluster)  [unwired: 1 in]
          n24 = Compound Arithmetic op=unknown(w104, 2 ("value")) -> (w95:i32)
          n25 = call "AlliGator Get Decay Fit Parameter Map Data.vi"("Multiple Decays Fit Parameters"=w51, "Compute Decay Fit Parameter Map"=w96, "Output ROI centers?"=w96, "X Resolution"=w84, "Y Resolution"=w83, "Error In"=w97, "Map index"=w95, "Selected ROI Array"=w43) -> ("Map Data (V x H)"=w82:dbl[][], "ROI Centers"=w81:cluster{"X":dbl, "Y":dbl}[], "Error Out"=w71:errorcluster)  [unwired: 3 in, 2 out]
          n26 = To Long Integer(number=w81) -> (32bit integer=w80:cluster{"X":i32, "Y":i32}[])
          n27 = call "Alligator Variables Storage.vi"("AlliGator Variable"=AlliGator_Variables_List."Source Image:ROIs" ("Alligator Variable"), "Error In"=w71) -> ("Error Out"=w92:errorcluster, "Data out"=w93:variant)  [unwired: 7 in, 1 out]
          n28 = call "IMAQ ImageToArray"("error in (no error)"=w71, "Image"=w73) -> ("Image Pixels (Float)"=w72:sgl[][], "error out"=w70:errorcluster)  [unwired: 2 in, 3 out]
          n29 = Variant To Data(error in=w92, type=T13[] [] ("ROIs"), Variant=w93) -> (data=w90:T13[], error out=w89:errorcluster)
          n30 = Array Max & Min(array=w72) -> (max value=w68:sgl, min value=w69:sgl)  [unwired: 2 out]
          n31 = for {
            tunnel: w90 -> [w197] mode=indexing
            tunnel: [w194] -> w88 mode=indexing
            tunnel: [w193] -> w85 mode=indexing
            shift-right: [w195] -> w86
            shift-left: w89 -> [w196]
            tunnel: [w192] -> w79 mode=indexing
            n32 = Unbundle By Name(w197) -> ("ROI Name"=w192:string, "ROI Descriptor"=w193:T14)
            n33 = call "ROI Barycenter.vi"("Error In"=w196, "ROI Descriptor in"=w193) -> ("Error Out"=w195:errorcluster, "Single Point ROI?"=w194:bool)  [unwired: 7 in, 1 out]
          }
          n34 = call "AlliGator Sliced Mean, SDV & CV Enter Data Dialog.vi"("Error In"=w70, "X min"=w69, "X max"=w68) -> ("Error Out"=w66:errorcluster, "Cancelled?"=w65:bool, "Slices Definition out"=w62:T53)  [unwired: 6 in]
          n35 = Bundle By Name(cluster=w62, "Output Abscissa Statistics Plots"=TRUE) -> (w47:T53)
          n36 = And Array Elements(Boolean array=w88) -> (logical AND=w63:bool)
          n37 = Or(x=w65, y=w63) -> (x .or. y?=w64:bool)
          n38 = Merge Errors(w66, w86) -> (w67:errorcluster)
          n39 = case shown="False" w64 {
            tunnel: [w135 w178] -> w87
            tunnel: w67 -> [w140 _]
            tunnel: w85 -> [w146 _]
            tunnel: w84 -> [w124 _]
            tunnel: w83 -> [w123 _]
            tunnel: w82 -> [w145 _]
            tunnel: w80 -> [w144 _]
            tunnel: w79 -> [w143 _]
            tunnel: w72 -> [w142 _]
            tunnel: w63 -> [_ w177]
            tunnel: w47 -> [w139 _]
            tunnel: [w131 w175] -> w57
            tunnel: [w134 w176] -> w56
            tunnel: w48 -> [w121 _]
            tunnel: w55 -> [w138 w175]
            tunnel: [w130 _] -> w54
            tunnel: w53 -> [w119 w176]
            tunnel: [w129 _] -> w52
            tunnel: w38 -> [w127 _]
            tunnel: [w120 _] -> w37
            frame False {
              # "Most ROIs are not single-pixel"
              n40 = for "For Loop on ROIs" {
                tunnel: w146 -> [w164] mode=indexing
                tunnel: w140 -> [w163]
                tunnel: w124 -> [w162]
                tunnel: w123 -> [w161]
                tunnel: w145 -> [w159]
                tunnel: w144 -> [w158]
                tunnel: w143 -> [w156] mode=indexing
                tunnel: w142 -> [w154]
                tunnel: [w152] -> w141 mode=indexing if=w149
                tunnel: [w147] -> w122 mode=indexing
                n41 = call "Create Single Pixel ROIs from ROI (Core).vi"("Y Resolution"=w161, "X Resolution"=w162, "error in (no error)"=w163, "ROI Descriptor"=w164) -> ("error out"=w151:errorcluster, "Point Array"=w160:cluster{"Numeric":i32, "Numeric":i32}[])  [unwired: 5 in, 1 out]
                n42 = for "Looks for map data for every pixel in ROI" {
                  tunnel: w160 -> [w170] mode=indexing
                  tunnel: w159 -> [w173]
                  tunnel: w158 -> [w174]
                  tunnel: [w172] -> w157 mode=indexing if=w167
                  tunnel: [w170] -> w155 mode=indexing if=w167
                  tunnel: w154 -> [w169]
                  tunnel: [w168] -> w148 mode=indexing if=w167
                  n43 = Search 1D Array(1D array=w174, element=w170) -> (index of element=w171:i32)  [unwired: 1 in]
                  n44 = Unbundle(w170) -> ("Numeric"=w166:i32, "Numeric"=w165:i32)
                  n45 = Greater Or Equal To 0?(x=w171) -> (x >= 0?=w167:bool)
                  n46 = Index Array(array=w173, index (row)=w165, index (col)=w166) -> (element=w172:dbl)
                  n47 = Index Array(array=w169, index (row)=w165, index (col)=w166) -> (element=w168:sgl)
                }
                n48 = Bundle By Name(cluster=T17 {"ROI Name"="", "Intensity Array"=[], "Lifetime Array"=[], "Coordinate Array"=[], "I Slice Bin Boundaries"=[], "Sliced <tau>"=[], "Sliced SDV(<tau>)"=[], "Sliced CV(<tau>)"=[], "Sliced #Elements"=[], "I Slice <I>"=[], "Sliced CV SDV(<tau>)"=[]}, "ROI Name"=w156, "Intensity Array"=w148, "Lifetime Array"=w157, "Coordinate Array"=w155) -> (w152:T17)
                n49 = Add Array Elements(numeric array=w148) -> (sum=w147:sgl)
                n50 = Unbundle By Name(w151) -> ("status"=w150:bool)
                n51 = Not(x=w150) -> (.not. x?=w149:bool)
              }
              n52 = call "AlliGator Compute Lifetime Variances.vi"("error in (no error)"=w140, "Lifetime Variance Data Array (in)"=w141, "Slices Definition"=w139) -> ("error out"=w137:errorcluster, "Parameter Map Names"=w129:string[], "Lifetime Variance Data Array (out)"=w136:T17[])  [unwired: 6 in]
              n53 = call "AlliGator Compute Lifetime Variance Map (Core).vi"("Build New Maps"=TRUE, "Function Parameters"=w127, "error in (no error)"=w137, "Lifetime Variance Data Array"=w136) -> ("error out"=w125:errorcluster, "CV Bootstrap SDV Test kappa x SDV"=w116:dbl, "CV Residual Test kappa x SDV"=w117:dbl, "Maps Data"=w126:dbl[][])  [unwired: 4 in]
              n54 = Format Into String(format string="(CV Res. x k = %#g, CV Boot. SDV x k = %#g)", initial string=w121, w117, w116) -> (resulting string=w120:string)  [unwired: 1 in, 1 out]
              n55 = call "Check for Names v2.vi"("New Name"=w120, "Name List"=w138, "Error In"=w125) -> ("New Name List"=w131:string[], "New Name"=w130:string, "Error Out"=w135:errorcluster)  [unwired: 3 in, 1 out]
              n56 = Bundle By Name(cluster=T16 {"Map Set Name"="", "[Parameter Names]"=[], "[[Parameters]]"=[], "[[Parameter SDVs]]"=[], "Decay Array Time Axis"=[], "[[IRFs]]"=[], "IRF Array Time Axis"=[], "X Resolution"=0, "Y Resolution"=0, "Intensity Array"=[]} ("[Parameter Maps]"), "[Parameter Names]"=w129, "[[Parameters]]"=w126, "Map Set Name"=w130, "X Resolution"=w124, "Y Resolution"=w123, "Intensity Array"=w122) -> (w133:T16)
              n57 = Build Array (concatenate)(w119, w133) -> (w134:T16[])
            }
            frame True {
              # "All single-pixel ROIs: can't compute ROI variance"
              n58 = case shown="True" w177 {
                tunnel: [w179 w185] -> w178
                frame False {
                  n59 = xnode "Error Ring"() -> ("error out"=w179:errorcluster)
                }
                frame True {
                  n60 = xnode "Error Ring"() -> ("error out"=w185:errorcluster)
                  n61 = One Button Dialog(message="Lifetime variance analysis requires ROIs with a minimum of points.\nAll ROIs are currently single-pixel ROIs.\nPlease clear the current single-pixel ROIs and load multi-pixel ones.") -> ()  [unwired: 1 in, 1 out]
                }
              }
            }
          }
          n62 = in-place-cluster #2("Single Data Point Path"=w61, "[Time-Series Paths]"=w60, "Current Dataset"=w59, "[[Multiple Decays Fit Parameters]]"=w51, "[Decay Fit Parameter Names]"=w58, "Current Dataset Images 1.SGL Sum Image"=w50, "Current Dataset Images 2.SGL Sum Image"=w49, "[Map Set Names]"=w57, "[Parameter Maps]"=w56, "Selected ROIs Array"=w43) -> (w33:T18)
        }
        n63 = in-place-dvr #1(w33) -> (w24:refnum<data-value>)  [unwired: 1 out]
      }
      n64 = call "High Resolution Timing.vi"("relative seconds (NaN)"=w19, "Error In"=w16) -> ("elapsed (relative) seconds"=w12:dbl, "Error Out"=w14:errorcluster)  [unwired: 15 in, 1 out]
      n65 = Format Into String(format string="\nCPU: %#g s", initial string=w20, error in=w14, w12) -> (resulting string=w15:string, error out=w13:errorcluster)
    }
    frame Error {
    }
  }
  "error out" <- w7
  "AlliGator IV DVR out" <- w9
  "Message" <- w4
  "CPU (s)" <- w3
  "New Parameter Set Name" <- w2
  "Parameter Map Names" <- w1
